vi "Read Listbox Header.vi"(8 "error in":errorcluster, 11 "Listbox Ref in":refnum<vi>) -> (0 "error out":errorcluster, 1 "Value":string, 2 "Interpret As Unicode":bool, 3 "Listbox Ref out":refnum<vi>)   [LabVIEW 2020, in "G-Unicode.lvlib"]
uses:
  G-Unicode.lvlib
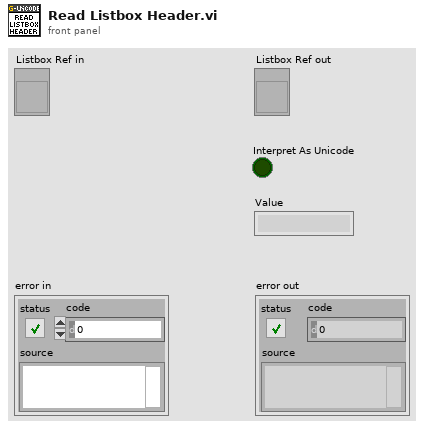
[diagram p1: front panel]
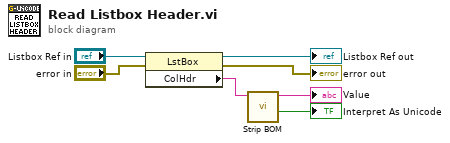
[diagram p0: block diagram]
diagram:
  n1 = property class="LstBox"(reference="Listbox Ref in", error in="error in") -> (reference out=→"Listbox Ref out":refnum<vi>, error out=→"error out":errorcluster, "ColHdr"=w3:string)
  n2 = call "Strip BOM.vi"("String"=w3) -> ("BOM Found"=→"Interpret As Unicode":bool, "String without BOM"=→"Value":string)  [unwired: 8 in, 1 out]
